vi "loadAndRun.vi"(3 "error in (no error)":errorcluster, 5 "path":path) -> (0 "error out":errorcluster, 2 "vi refnum out":refnum<vi>)   [LabVIEW 2011, in "ttmServer.lvclass"]
doc: "Opens a refnum to the specified VI and, optionally, runs it."
uses:
  ttmServer.lvclass
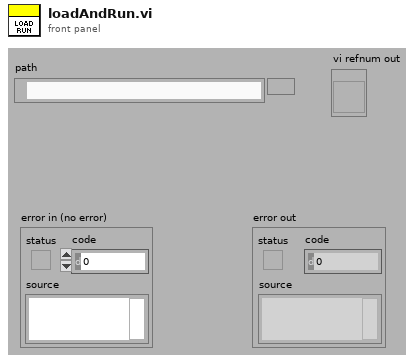
[diagram p1: front panel]
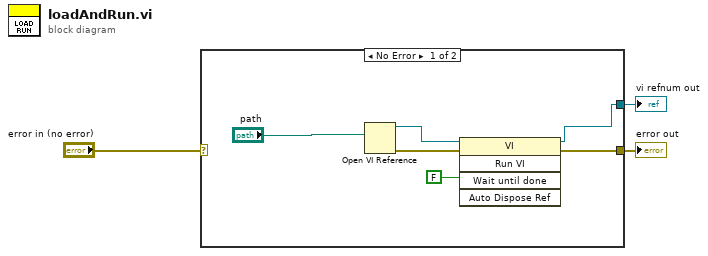
[diagram p0: block diagram]
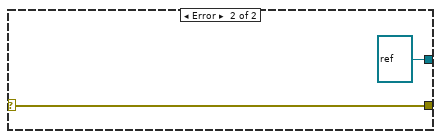
[diagram p2: hidden frame]
diagram:
  n1 = case shown="No Error" "error in (no error)" {
    selector: "error in (no error)" -> [_ w10]
    tunnel: [w8 refnum<vi> refnum] -> w2
    tunnel: [w6 w10] -> w1
    frame No Error {
      n2 = Open VI Reference(vi path="path") -> (vi reference=w9:refnum<vi>, error out=w7:errorcluster)  [unwired: 5 in]
      n3 = invoke class="VI" method="Run VI"(reference=w9, error in=w7, "Wait until done"=FALSE) -> (reference out=w8:refnum<vi>, error out=w6:errorcluster)  [unwired: 2 in, 3 out]
    }
    frame Error {
    }
  }
  "vi refnum out" <- w2
  "error out" <- w1
